vi "Open Demo.vi"(7 "Stop Demo":refnum<user-event>, 8 "error in":errorcluster, 10 "VI":refnum<vi>, 11 "Main Subpanel":refnum<vi>) -> (0 "error out":errorcluster)   [LabVIEW 2020]
uses:
  <vilib>/Utility/miscctls.llb/LVPointTypeDef.ctl
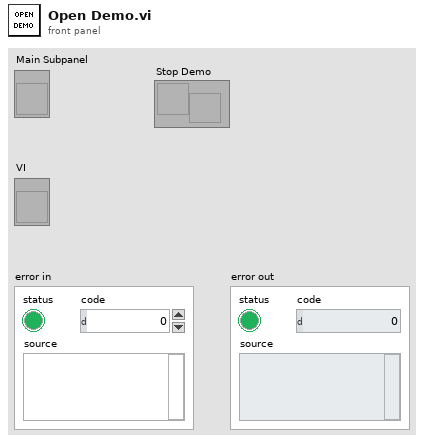
[diagram p1: front panel]
types:
  T1 = typedef "LVPointTypeDef.ctl" = cluster{"Horizontal":i16, "Vertical":i16}
  T2 = typedef "LVBoundsTypeDef.ctl" = cluster{"Width":u32, "Height":u32}
  T3 = typedef "LVRectTypeDef.ctl" = cluster{"Left":i16, "Top":i16, "Right":i16, "Bottom":i16}
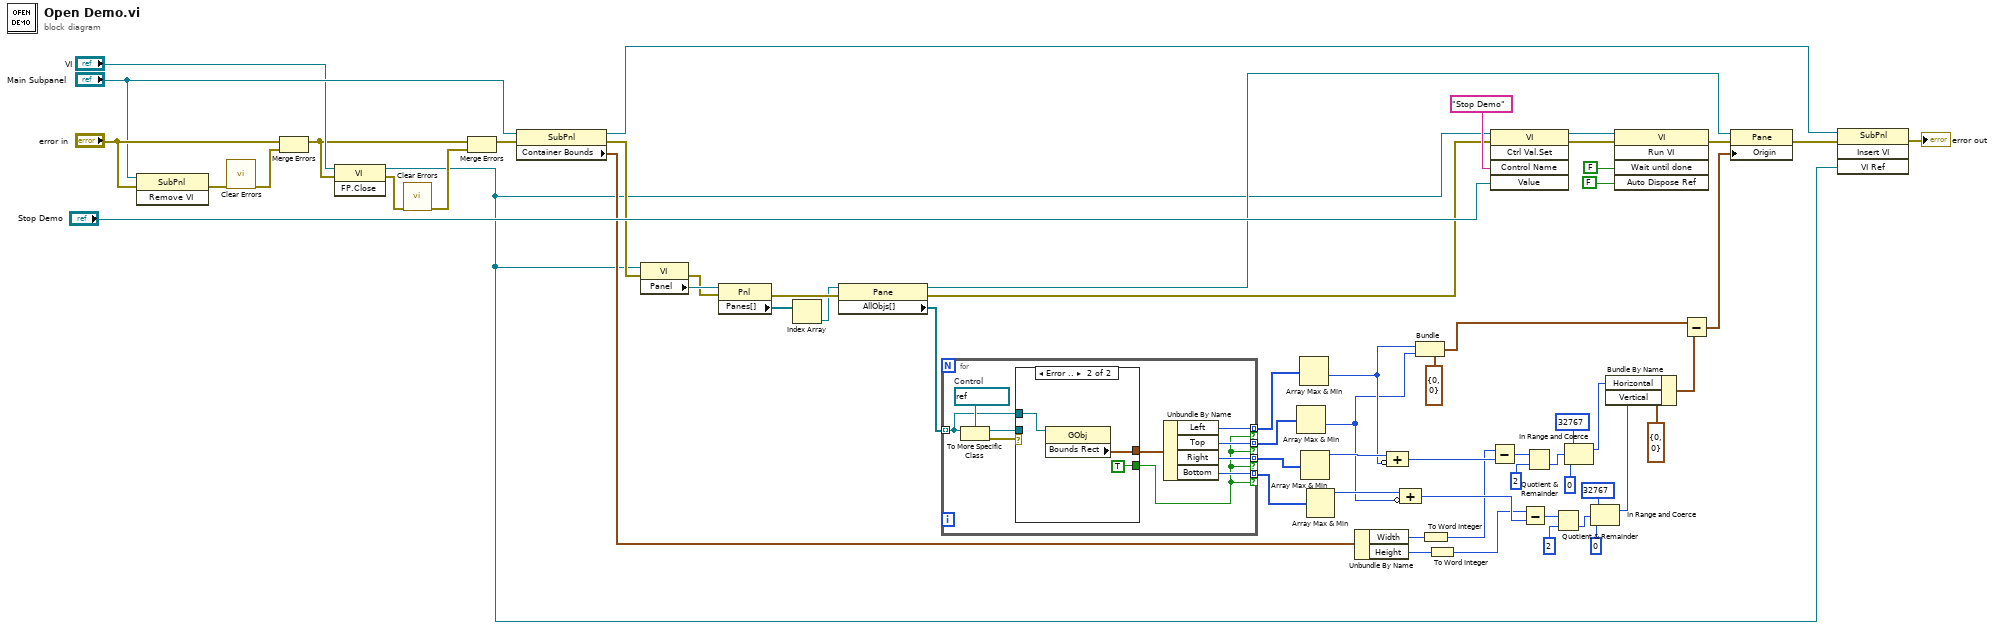
[diagram p0: block diagram]
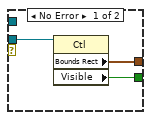
[diagram p2: hidden frame]
diagram:
  n1 = invoke class="SubPnl" method="Remove VI"(reference="Main Subpanel", error in="error in") -> (error out=w56:errorcluster)  [unwired: 1 in, 2 out]
  n2 = call <vilib>:"Clear Errors.vi"("error in (no error)"=w56) -> ("error out"=w55:errorcluster)  [unwired: 5 in, 1 out]
  n3 = Merge Errors("error in", w55) -> (w5:errorcluster)
  n4 = invoke class="VI" method="FP.Close"(reference="VI", error in=w5) -> (reference out=w1:refnum<vi>, error out=w7:errorcluster)  [unwired: 1 in, 1 out]
  n5 = call <vilib>:"Clear Errors.vi"("error in (no error)"=w7) -> ("error out"=w6:errorcluster)  [unwired: 5 in, 1 out]
  n6 = Merge Errors(w5, w6) -> (w4:errorcluster)
  n7 = property class="SubPnl"(reference="Main Subpanel", error in=w4) -> (reference out=w3:refnum<vi>, error out=w16:errorcluster, "Container Bounds"=w15:T2)
  n8 = property class="VI"(reference=w1, error in=w16) -> (error out=w46:errorcluster, "Panel"=w48:refnum<vi>)  [unwired: 1 out]
  n9 = property class="Pnl"(reference=w48, error in=w46) -> (error out=w45:errorcluster, "Panes[]"=w47:refnum<vi>[])  [unwired: 1 out]
  n10 = Index Array(array=w47) -> (element=w44:refnum<vi>)  [unwired: 1 in]
  n11 = property class="Pane"(reference=w44, error in=w45) -> (reference out=w14:refnum<vi>, error out=w13:errorcluster, "AllObjs[]"=w43:refnum<vi>[])
  n12 = for {
    tunnel: w43 -> [w68] mode=indexing
    tunnel: [w66] -> w42 mode=indexing if=w62
    tunnel: [w65] -> w41 mode=indexing if=w62
    tunnel: [w64] -> w40 mode=indexing if=w62
    tunnel: [w63] -> w39 mode=indexing if=w62
    w70 = refnum<vi> refnum  # Control
    n13 = To More Specific Class(target class=w70, reference=w68) -> (specific class reference=w71:refnum<vi>, error out=w69:errorcluster)  [unwired: 1 in]
    n14 = case shown="Error .." w69 {
      tunnel: w71 -> [w74 _]
      tunnel: w68 -> [_ w77]
      tunnel: [w73 w76] -> w67
      tunnel: [w72 TRUE] -> w62
      frame No Error {
        n15 = property class="Ctl"(reference=w74) -> ("Bounds Rect"=w73:T3, "Visible"=w72:bool)  [unwired: 1 in, 2 out]
      }
      frame Error {
        n16 = property class="GObj"(reference=w77) -> ("Bounds Rect"=w76:T3)  [unwired: 1 in, 2 out]
      }
    }
    n17 = Unbundle By Name(w67) -> ("Left"=w66:i16, "Top"=w65:i16, "Right"=w64:i16, "Bottom"=w63:i16)
  }
  n18 = Array Max & Min(array=w41) -> (min value=w10:i16)  [unwired: 3 out]
  n19 = Array Max & Min(array=w42) -> (min value=w11:i16)  [unwired: 3 out]
  n20 = Array Max & Min(array=w40) -> (max value=w38:i16)  [unwired: 3 out]
  n21 = Array Max & Min(array=w39) -> (max value=w37:i16)  [unwired: 3 out]
  n22 = Unbundle By Name(w15) -> ("Width"=w33:u32, "Height"=w26:u32)
  n23 = Compound Arithmetic op=ADD(w38, invert w11) -> (w34:i16)
  n24 = Compound Arithmetic op=ADD(w37, invert w10) -> (w25:i16)
  n25 = Bundle(cluster=T1 {"Horizontal"=0, "Vertical"=0} ("Origin"), "Horizontal"=w11, "Vertical"=w10) -> (w9:T1)
  n26 = To Word Integer(number=w33) -> (16bit integer=w23:i16)
  n27 = To Word Integer(number=w26) -> (16bit integer=w22:i16)
  n28 = Subtract(x=w23, y=w34) -> (x-y=w32:i16)
  n29 = invoke class="VI" method="Ctrl Val.Set"(reference=w1, error in=w13, "Control Name"="Stop Demo", "Value"="Stop Demo") -> (reference out=w51:refnum<vi>, error out=w54:errorcluster)  [unwired: 1 in, 3 out]
  n30 = Subtract(x=w22, y=w25) -> (x-y=w27:i16)
  n31 = Quotient & Remainder(x=w32, y=i16 2) -> (floor(x/y)=w20:i16)  [unwired: 1 out]
  n32 = Quotient & Remainder(x=w27, y=i16 2) -> (floor(x/y)=w19:i16)  [unwired: 1 out]
  n33 = In Range and Coerce(upper limit=i16 32767, x=w20, lower limit=i16 0) -> (coerced(x)=w29:i16)  [unwired: 1 out]
  n34 = In Range and Coerce(upper limit=i16 32767, x=w19, lower limit=i16 0) -> (coerced(x)=w24:i16)  [unwired: 1 out]
  n35 = Bundle By Name(cluster=T1 {"Horizontal"=0, "Vertical"=0} ("Origin"), "Horizontal"=w29, "Vertical"=w24) -> (w35:T1)
  n36 = invoke class="VI" method="Run VI"(reference=w51, error in=w54, "Wait until done"=FALSE ("Wait Until Done"), "Auto Dispose Ref"=FALSE ("Auto Dispose Reference")) -> (error out=w52:errorcluster)  [unwired: 1 in, 4 out]
  n37 = Subtract(x=w9, y=w35) -> (x-y=w12:T1)
  n38 = property class="Pane"(reference=w14, error in=w52, "Origin"=w12) -> (error out=w2:errorcluster)  [unwired: 1 out]
  n39 = invoke class="SubPnl" method="Insert VI"(reference=w3, error in=w2, "VI Ref"=w1) -> (error out=→"error out":errorcluster)  [unwired: 1 in, 3 out]
